vi "RT Driver VI.vi"(7 "Operation":T1, 11 "Device Reference in":T2 format="%.0x") -> (0 "Error Code":i32)   [LabVIEW 2017, in "Exercise 7.2 Engine.lvlib"]
uses:
  Exercise 7.2 Engine.lvlib
  <vilib>/NI Veristand/Custom Device API/Custom Device Item Ref.ctl
  <vilib>/NI Veristand/Custom Device API/Model Interface Driver VI Operation.ctl
  <vilib>/NI Veristand/Custom Device API/Custom Device Channel Type.ctl
  <vilib>/NI Veristand/Custom Device API/Data Reference.ctl
  <vilib>/NI Veristand/Custom Device API/Data Access Type.ctl
  <vilib>/NI Veristand/Custom Device API/Get Item Property (U16).vi
  <vilib>/NI Veristand/Custom Device API/Get Item Property (String).vi
  <vilib>/NI Veristand/Custom Device API/Global Data Refs.vi
  <vilib>/NI Veristand/Custom Device API/Custom Device API.lvlib
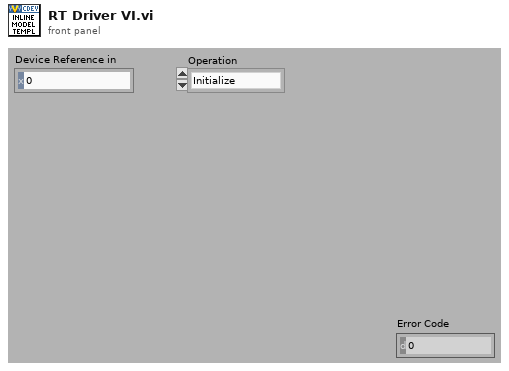
[diagram p1: front panel]
types:
  T1 = typedef "Custom Device API.lvlib/Model Interface Driver VI Operation.ctl" = enum16{"Initialize", "Start", "Execute Model", "Close"}
  T2 = typedef "Custom Device API.lvlib/Custom Device Item Ref.ctl" = u64
  T3 = typedef "Custom Device API.lvlib/Data Reference.ctl" = i32
  T4 = cluster{"Input Values":dbl[], "Input Refs":T3[], "Output Values":dbl[], "Output Refs":T3[], "Local Port":u16, "Remote Port":u16, "Address":string}
  T5 = typedef "Custom Device API.lvlib/Custom Device Channel Type.ctl" = enum16{"Input", "Output"}
  T6 = typedef "Custom Device API.lvlib/Data Access Type.ctl" = enum16{"Read", "Write"}
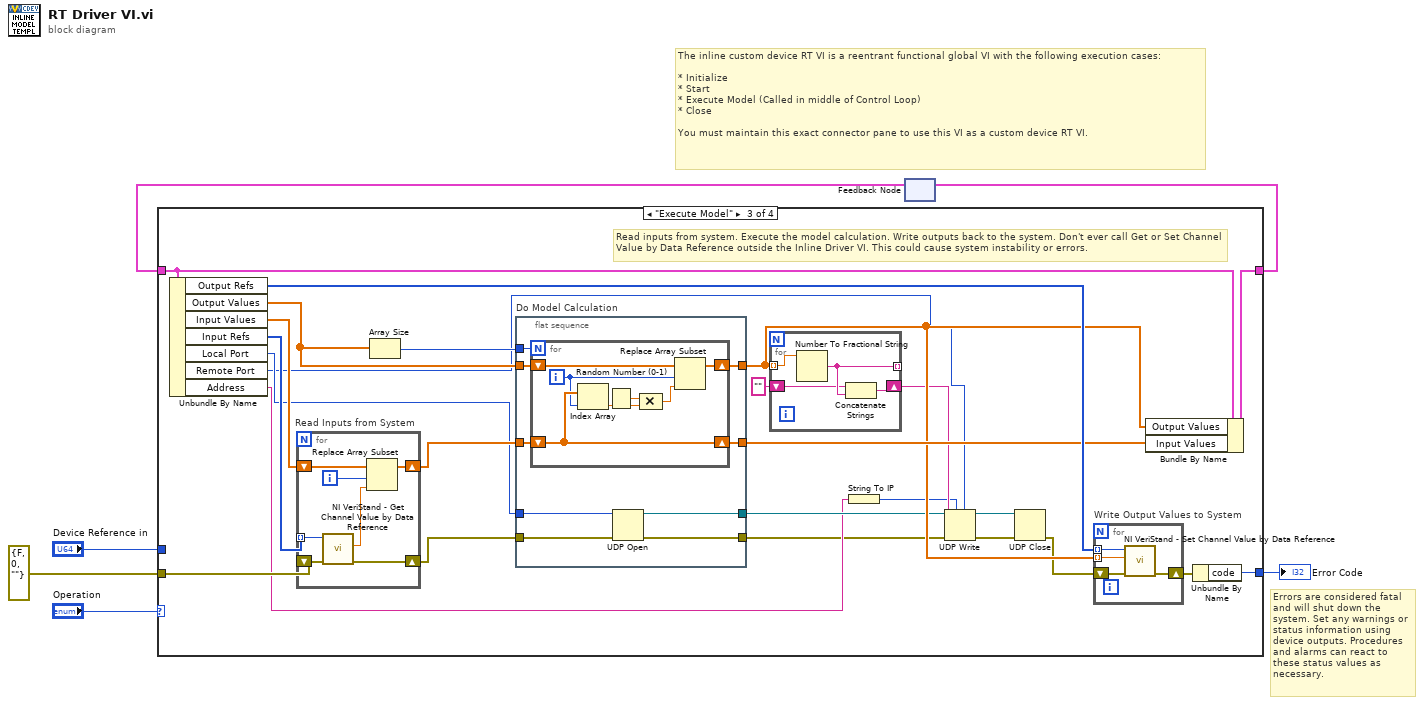
[diagram p0: block diagram]
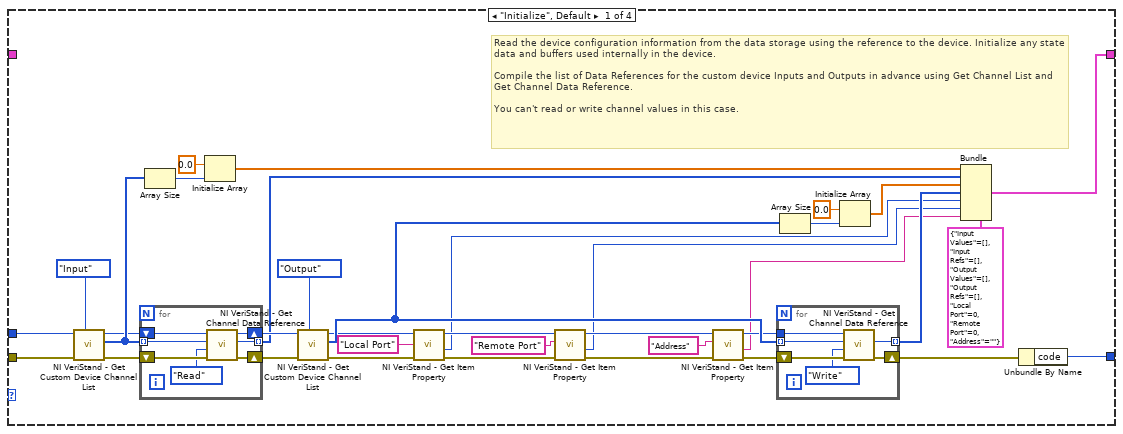
[diagram p2: hidden frame]
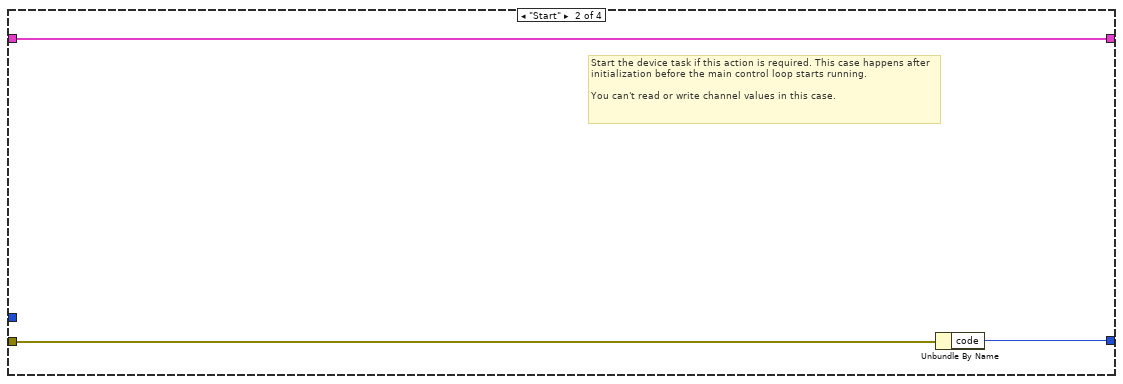
[diagram p3: hidden frame]
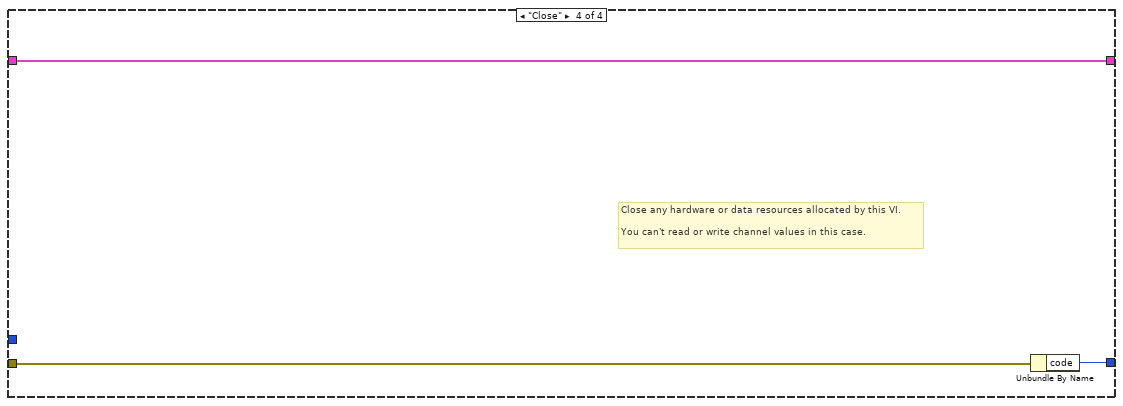
[diagram p4: hidden frame]
diagram:
  # "Errors are considered fatal and will shut down the system. Set any warnings or status information using device outputs. Procedures and alarms can react to these status values as necessary."
  # "The inline custom device RT VI is a reentrant functional global VI with the following execution cases:\n\n* Initialize\n* Start\n* Execute Model (Called in middle of Control Loop)\n* Close\n\nYou must maintain this exact connector pane to use this VI as a custom device RT VI."
  n1 = feedback #1() -> (w1:T4)  [unwired: 1 out]
  n2 = case shown="\"Execute Model\"" "Operation" {
    tunnel: [w23 w58 w77 w117] -> w5
    tunnel: w1 -> [_ w58 w78 w117]
    tunnel: "Device Reference in" -> [w24 _ _ _]
    tunnel: [w22 w56 w74 w116] -> w3
    tunnel: errorcluster {"status"=FALSE, "code"=0, "source"=""} ("error in (no error)") -> [w21 w57 w81 w115]
    frame "Initialize", Default {
      # "Read the device configuration information from the data storage using the reference to the device. Initialize any state data and buffers used internally in the device.\n\nCompile the list of Data References for the custom device Inputs and Outputs in advance using Get Channel List and Get Channel Data Reference.\n\nYou can't read or write channel values in this case."
      n3 = call <vilib>:"NI VeriStand - Get Custom Device Channel List.vi"("Channel Type"=Custom_Device_Channel_Type."Input", "error in (no error)"=w21, "Device Ref in"=w24) -> ("error out"=w30:errorcluster, "Specified Channel Ref List"=w31:T2[], "Device Ref out"=w29:T2)  [unwired: 6 out]
      n4 = for {
        shift-right: [w50] -> w42
        shift-left: w29 -> [w54]
        tunnel: w31 -> [w53] mode=indexing
        shift-right: [w51] -> w33
        shift-left: w30 -> [w55]
        tunnel: [w49] -> w34 mode=indexing
        n5 = call <vilib>:"NI VeriStand - Get Channel Data Reference.vi"("error in (no error)"=w55, "Access"=Data_Access_Type."Read", "Channel Ref in"=w53, "Device Ref in"=w54) -> ("error out"=w51:errorcluster, "Channel Data Reference"=w49:T3, "Device Ref out"=w50:T2)  [unwired: 5 out]
      }
      n6 = Array Size(array=w31) -> (size(s)=w26:i32)
      n7 = Initialize Array(0.0 ("element"), w26) -> (w25:dbl[])
      n8 = call <vilib>:"NI VeriStand - Get Custom Device Channel List.vi"("Channel Type"=Custom_Device_Channel_Type."Output", "error in (no error)"=w33, "Device Ref in"=w42) -> ("error out"=w12:errorcluster, "Specified Channel Ref List"=w37:T2[], "Device Ref out"=w13:T2)  [unwired: 6 out]
      n9 = call-poly <vilib>:"NI VeriStand - Get Item Property.vi"("error in (no error)"=w12, "Property Name"="Local Port", "Item Ref in"=w13) -> ("error out"=w17:errorcluster, "Value"=w9:u16, "Item Ref out"=w20:T2)  [unwired: 5 in, 1 out]
      n10 = call-poly <vilib>:"NI VeriStand - Get Item Property.vi"("error in (no error)"=w17, "Property Name"="Remote Port", "Item Ref in"=w20) -> ("error out"=w18:errorcluster, "Value"=w8:u16, "Item Ref out"=w19:T2)  [unwired: 5 in, 1 out]
      n11 = call-poly <vilib>:"NI VeriStand - Get Item Property.vi"("error in (no error)"=w18, "Property Name"="Address", "Item Ref in"=w19) -> ("error out"=w11:errorcluster, "Value"=w7:string, "Item Ref out"=w10:T2)  [unwired: 5 in, 1 out]
      n12 = for {
        tunnel: w37 -> [w46] mode=indexing
        shift-right: [w44] -> w40
        shift-left: w11 -> [w48]
        tunnel: [w43] -> w39 mode=indexing
        tunnel: w10 -> [w47]
        n13 = call <vilib>:"NI VeriStand - Get Channel Data Reference.vi"("error in (no error)"=w48, "Access"=Data_Access_Type."Write", "Channel Ref in"=w46, "Device Ref in"=w47) -> ("error out"=w44:errorcluster, "Channel Data Reference"=w43:T3)  [unwired: 6 out]
      }
      n14 = Array Size(array=w37) -> (size(s)=w36:i32)
      n15 = Initialize Array(0.0 ("element"), w36) -> (w38:dbl[])
      n16 = Bundle(cluster=T4 {"Input Values"=[], "Input Refs"=[], "Output Values"=[], "Output Refs"=[], "Local Port"=0, "Remote Port"=0, "Address"=""}, "Input Values"=w25, "Input Refs"=w34, "Output Values"=w38, "Output Refs"=w39, "Local Port"=w9, "Remote Port"=w8, "Address"=w7) -> (w23:T4)
      n17 = Unbundle By Name(w40) -> ("code"=w22:i32)
    }
    frame "Start" {
      # "Start the device task if this action is required. This case happens after initialization before the main control loop starts running.\n\nYou can't read or write channel values in this case."
      n18 = Unbundle By Name(w57) -> ("code"=w56:i32)
    }
    frame "Execute Model" {
      # "Read inputs from system. Execute the model calculation. Write outputs back to the system. Don't ever call Get or Set Channel Value by Data Reference outside the Inline Driver VI. This could cause system instability or errors."
      n19 = Unbundle By Name(w78) -> ("Output Refs"=w76:T3[], "Output Values"=w72:dbl[], "Input Values"=w83:dbl[], "Input Refs"=w82:T3[], "Local Port"=w68:u16, "Remote Port"=w63:u16, "Address"=w62:string)
      n20 = for "Read Inputs from System" {
        shift-right: [w104] -> w79
        shift-left: w81 -> [w110]
        tunnel: w82 -> [w109] mode=indexing
        shift-right: [w107] -> w80
        shift-left: w83 -> [w108]
        i -> [w106]
        n21 = call <vilib>:"NI VeriStand - Get Channel Value by Data Reference.vi"("error in (no error)"=w110, "Data Reference in"=w109) -> ("error out"=w104:errorcluster, "Value"=w105:dbl)  [unwired: 8 out]
        n22 = Replace Array Subset(array=w108, new element=w105, index=w106) -> (w107:dbl[])
      }
      n23 = Array Size(array=w72) -> (size(s)=w71:i32)
      n24 = flat-sequence "Do Model Calculation" {
        tunnel: w80 -> [w95]
        tunnel: w79 -> [w90]
        tunnel: w72 -> [w96]
        tunnel: [w94] -> w73
        tunnel: [w93] -> w70
        tunnel: [w89] -> w60
        tunnel: w71 -> [w92]
        tunnel: w68 -> [w91]
        tunnel: [w88] -> w66
        frame #0 {
          n25 = for {
            N: w92 -> [_]
            shift-right: [w102] -> w93
            shift-left: w96 -> [w103]
            shift-right: [w99] -> w94
            shift-left: w95 -> [w99]
            i -> [w97]
            n26 = Index Array(array=w99, index=w97) -> (element=w98:dbl)
            n27 = Random Number (0-1)() -> (number: 0 to 1=w101:dbl)
            n28 = Compound Arithmetic op=MULTIPLY(w101, w98) -> (w100:dbl)
            n29 = Replace Array Subset(array=w103, new element=w100, index=w97) -> (w102:dbl[])
          }
          n30 = UDP Open(8:w90, 11:w91) -> (port=w88:refnum<k16>, 0:w89:errorcluster)  [unwired: 3 in, 1 out]
        }
      }
      n31 = for {
        tunnel: w70 -> [w87] mode=indexing
        tunnel: [w86] -> _ mode=indexing
        shift-right: [w85] -> w67
        shift-left: "" -> [w84]
        n32 = Number To Fractional String(number=w87) -> (F-format string=w86:string)  [unwired: 3 in]
        n33 = Concatenate Strings(w84, w86) -> (w85:string)
      }
      n34 = String To IP(1:w62) -> (0:w61:u32)
      n35 = UDP Write(address=w61, port or service name=w63, connection ID=w66, data in=w67, 8:w60) -> (error out=w65:errorcluster, 3:w64:refnum<k16>)  [unwired: 1 in]
      n36 = UDP Close(connection ID=w64, 8:w65) -> (error out=w59:errorcluster)  [unwired: 1 out]
      n37 = for "Write Output Values to System" {
        shift-right: [w113] -> w75
        shift-left: w59 -> [w114]
        tunnel: w70 -> [w112] mode=indexing
        tunnel: w76 -> [w111] mode=indexing
        n38 = call <vilib>:"NI VeriStand - Set Channel Value by Data Reference.vi"("error in (no error)"=w114, "Value"=w112, "Data Reference in"=w111) -> ("error out"=w113:errorcluster)  [unwired: 8 out]
      }
      n39 = Bundle By Name(cluster=w78, "Output Values"=w70, "Input Values"=w73) -> (w77:T4)
      n40 = Unbundle By Name(w75) -> ("code"=w74:i32)
    }
    frame "Close" {
      # "Close any hardware or data resources allocated by this VI.\n\nYou can't read or write channel values in this case."
      n41 = Unbundle By Name(w115) -> ("code"=w116:i32)
    }
  }
  "Error Code" <- w3
  n42 = feedback-in #1(w5) -> ()
